vi "Handle.vi"(8 "error in (no error)":errorcluster, 10 "Zero Timeout Message Handler in":refnum<class "Zero Timeout Message Handler.lvclass">, 11 "Message in":refnum<class "Poll Msg.lvclass">) -> (0 "error out":errorcluster, 2 "Zero Timeout Message Handler out":refnum<class "Zero Timeout Message Handler.lvclass">)   [LabVIEW 2024, in "Zero Timeout Message Handler.lvlib" / "Poll Msg.lvclass"]
uses:
  Poll Msg.lvclass
  Zero Timeout Message Handler/Zero Timeout Message Handler.lvclass
  Poll Msg.lvclass/Poll Msg.ctl
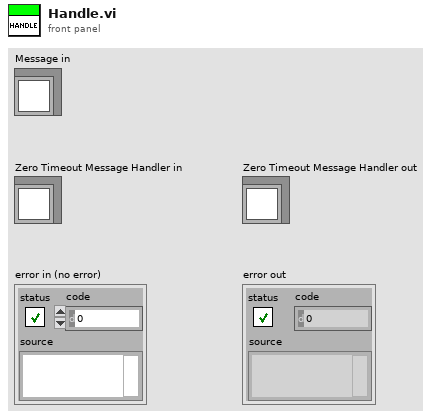
[diagram p1: front panel]
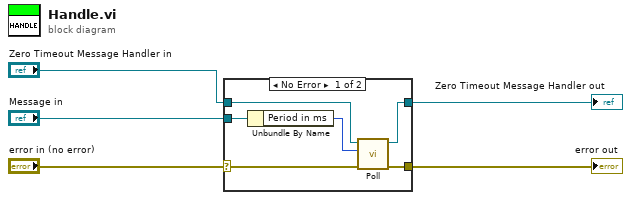
[diagram p0: block diagram]
diagram:
  n1 = case shown="No Error" "error in (no error)" {
    selector: "error in (no error)" -> [w8 w12]
    tunnel: "Zero Timeout Message Handler in" -> [w11 w13]
    tunnel: [w10 w13] -> w4
    tunnel: [w9 w12] -> w2
    tunnel: "Message in" -> [w7 _]
    frame No Error {
      n2 = Unbundle By Name(w7) -> ("Period in ms"=w6:u32)
      n3 = call-dynamic "Poll.vi"("error in (no error)"=w8, "Period in ms"=w6, "Zero Timeout Message Handler in"=w11) -> ("error out"=w9:errorcluster, "Zero Timeout Message Handler out"=w10:refnum<class "Zero Timeout Message Handler.lvclass">)  [unwired: 7 in]
    }
    frame Error {
    }
  }
  "error out" <- w2
  "Zero Timeout Message Handler out" <- w4
